vi "Process_And_Aim.vi"() -> (0 "Found Target":bool, 1 "Elevation Angle":dbl, 2 "Target Dist":dbl, 3 "Offset Angle From Perpendicular":dbl, 4 "Bounding Rect":T1)   [LabVIEW 2012]
panel:
  out "Angle Error":dbl
  out "Processed Image Out":T2(plugin-control)
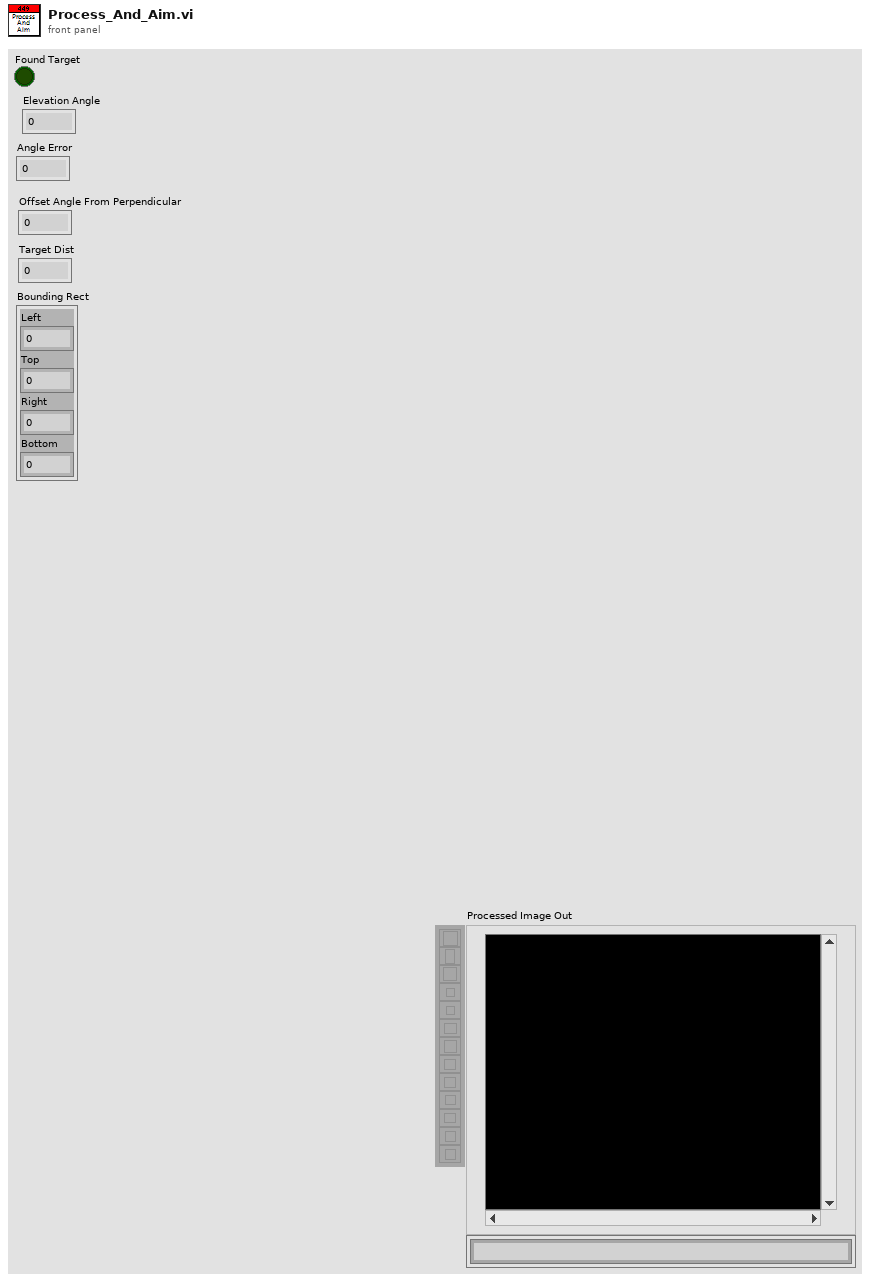
[diagram p1: front panel]
types:
  T1 = cluster{"Left":dbl, "Top":dbl, "Right":dbl, "Bottom":dbl}
  T2 = typedef "IMAQ Image.ctl" = refnum<image>
  T3 = cluster{"Image Out Light":T2, "Image Out Light":T2}
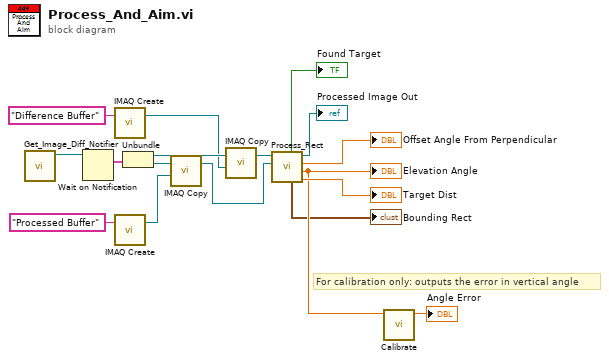
[diagram p0: block diagram]
diagram:
  # "For calibration only: outputs the error in vertical angle"
  n1 = call "Get_Image_Diff_Notifier.vi"() -> ("notifier out"=w10:refnum<notifier>)  [unwired: 11 in]
  n2 = Wait on Notification(notifier=w10) -> (notification=w9:T3)  [unwired: 3 in, 3 out]
  n3 = call "IMAQ Create"("Image Name"="Difference Buffer") -> ("New Image"=w7:T2)  [unwired: 4 in, 1 out]
  n4 = call "IMAQ Create"("Image Name"="Processed Buffer") -> ("New Image"=w2:T2)  [unwired: 4 in, 1 out]
  n5 = Unbundle(w9) -> ("Image Out Light"=w8:T2, "Image Out Light"=w3:T2)
  n6 = call "IMAQ Copy"("Image Dst"=w2, "Image Src"=w3) -> ("Image Dst Out"=w1:T2)  [unwired: 4 in, 1 out]
  n7 = call "IMAQ Copy"("Image Dst"=w7, "Image Src"=w8) -> ("Image Dst Out"=w6:T2)  [unwired: 4 in, 1 out]
  n8 = call "Process_Rect.vi"("Image to process"=w1, "Difference image"=w6) -> ("Target Dist"=→"Target Dist":dbl, "Vertical Angle"=w13:dbl, "Horizontal Angle"=→"Offset Angle From Perpendicular":dbl, "Processed Image Out"=→"Processed Image Out":T2, "Bounding Rect"=→"Bounding Rect":T1, "Found Target"=→"Found Target":bool)  [unwired: 4 in]
  "Elevation Angle" <- w13
  n9 = call "Calibrate.vi"("Calculated Vertical Angle"=w13) -> ("Vertical Angle Error"=→"Angle Error":dbl)  [unwired: 10 in]
